vi "LS_372_set_excitation.vi"(6 "Temperature":dbl, 7 "LS_Excitation old":dbl) -> (2 "Change of Excitation?":bool, 3 "LS_Excitation new":dbl)   [LabVIEW 2019]
panel:
  out "Path":path
  out "Excitation parameter":string(combo)
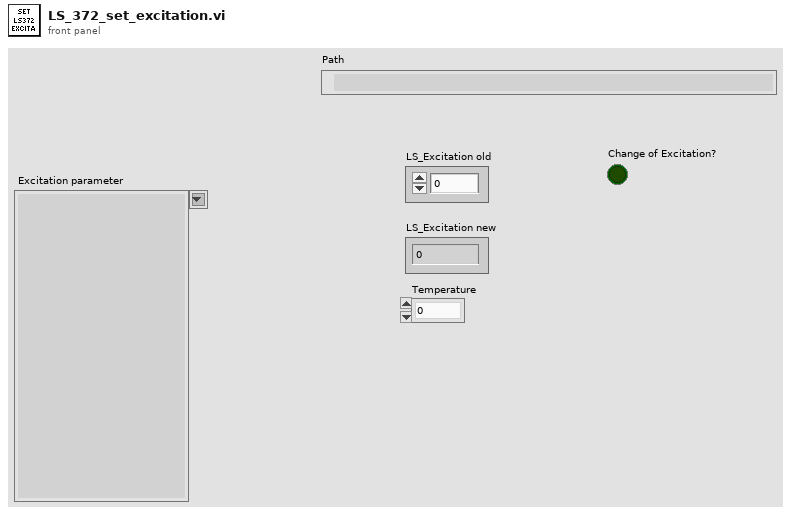
[diagram p1: front panel]
types:
  T1 = enum16{"open", "replace", "create", "open or create", "replace or create", "replace or create with confirmation"}
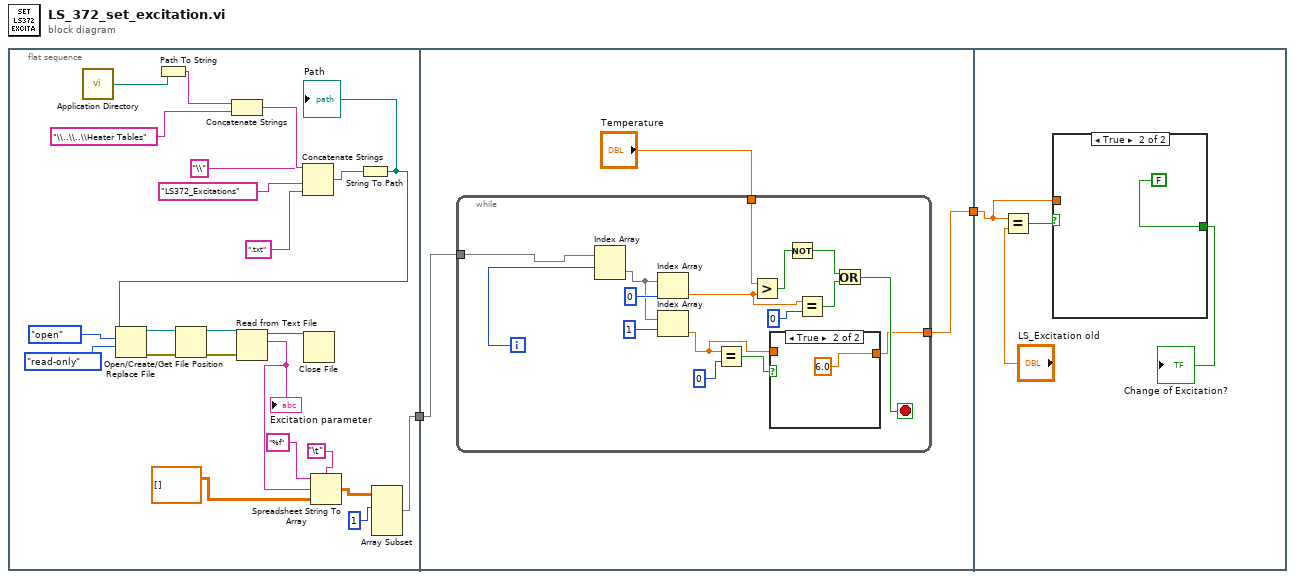
[diagram p0: block diagram]
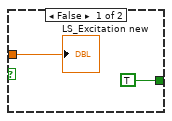
[diagram p3: hidden frame]
diagram:
  n1 = flat-sequence {
    tunnel: [w4] -> w2
    tunnel: w2 -> [w28]
    tunnel: [w27] -> w1
    tunnel: w1 -> [w48]
    frame #0 {
      n2 = call <vilib>:"Application Directory.vi"() -> ("Application Directory"=w25:path)
      n3 = Path To String(path=w25) -> (string=w24:string)
      n4 = Concatenate Strings(w24, "\\..\\..\\Heater Tables") -> (w22:string)
      n5 = Concatenate Strings(w22, "\\", "LS372_Excitations", ".txt") -> (w19:string)
      n6 = String To Path(string=w19) -> (path=w10:path)
      "Path" <- w10
      n7 = Open/Create/Replace File(file path (use dialog)=w10, operation (0:open)=T1."open", access (0:read/write)=enum16{"read/write", "read-only", "write-only"}."read-only") -> (refnum out=w15:refnum<file>, error out=w14:errorcluster)  [unwired: 3 in, 1 out]
      n8 = Get File Position(4:w14, 7:w15) -> (0:w12:errorcluster, 3:w13:refnum<file>)  [unwired: 1 out]
      n9 = Read from Text File(file (use dialog)=w13, error in=w12) -> (refnum out=w11:refnum<file>, text=w9:string)  [unwired: 2 in, 2 out]
      "Excitation parameter" <- w9
      n10 = Close File(refnum=w11) -> ()  [unwired: 1 in, 2 out]
      n11 = Spreadsheet String To Array(delimiter (Tab)="\t", format string="%f", spreadsheet string=w9, array type (2D Dbl)=dbl[][] []) -> (array=w5:dbl[][])
      n12 = Array Subset(array=w5, index (row)=1) -> (w4:dbl[][])  [unwired: 3 in]
    }
    frame #1 {
      n13 = while {
        tunnel: w28 -> [w44]
        tunnel: [w29] -> w27
        tunnel: "Temperature" -> [w39]
        i -> [w43]
        stop <- w33 stop-if-true
        n14 = Index Array(array=w44, index (row)=w43) -> (element=w40:dbl[])  [unwired: 1 in]
        n15 = Index Array(array=w40, index=0) -> (element=w35:dbl)
        n16 = Index Array(array=w40, index=1) -> (element=w30:dbl)
        n17 = Equal?(x=w30, y=0) -> (x = y?=w31:bool)
        n18 = Greater?(x=w39, y=w35) -> (0:w38:bool)
        n19 = case shown="True" w31 {
          tunnel: [w45 6.0] -> w29
          tunnel: w30 -> [w45 _]
          frame False {
          }
          frame True {
          }
        }
        n20 = Not(x=w38) -> (.not. x?=w37:bool)
        n21 = Equal?(x=w35, y=0) -> (x = y?=w36:bool)
        n22 = Or(x=w37, y=w36) -> (x .or. y?=w33:bool)
      }
    }
    frame #2 {
      n23 = Equal?(x=w48, y="LS_Excitation old") -> (x = y?=w49:bool)
      n24 = case shown="True" w49 {
        tunnel: w48 -> [w52 _]
        tunnel: [TRUE FALSE] -> w47
        frame False {
          "LS_Excitation new" <- w52
        }
        frame True {
        }
      }
      "Change of Excitation?" <- w47
    }
  }
